vi "(RAG) Retrieve Contexts from KB.vi"(0 "Python Session Refnum in":refnum<k35>, 1 "Chroma Database Folder":path, 5 "Knowledge Base Name":string, 7 "RAG Query":string="NI 9225的最高和最低电压是多少？它的售价是多少？", 9 "K":u32=5, 11 "error in":errorcluster, 12 "Embedding Model URL":string, 13 "Embedding Model Name":string) -> (4 "Python Session Refnum out":refnum<k35>, 6 "Retrieved Contexts":string="??????∵??????? ?Ё? RoHS\n\n\n\nЁ??? National Instruments ??Ё????? ??Ё???????????? (RoHS)??? National Instruments Ё? RoHS ????????? ni.com/environment/rohs_china? (For information about China RoHS compliance, go to ni.com/ environment/rohs_china.)\n\nCalibration\n\nYou can obtain the calibration certificate and information about calibration services for the NI 9225 at ni.com/calibration.\n\nCalibration interval . 1 year\n\nWorldwide Support and Services\n??????∵??????? ?Ё? RoHS\n\n\n\nЁ??? National Instruments ??Ё????? ??Ё???????????? (RoHS)??? National Instruments Ё? RoHS ????????? ni.com/environment/rohs_china? (For information about China RoHS compliance, go to ni.com/ environment/rohs_china.)\n\nCalibration\n\nYou can obtain the calibration certificate and information about calibration services for the NI 9225 at ni.com/calibration.\n\nCalibration interval . 1 year\n\nWorldwide Support and Services\nSafety Guidelines for Hazardous Locations\n\nThe NI 9225 is suitable for use in Class I, Div 2, Gr A, B, C, D, T4 and Class I, Zn 2, Gr IIC, T4 hazardous locations, and nonhazardous locations only. Follow these guidelines if you are installing the NI 9225 in a potentially explosive environment. Not following these guidelines may result in serious injury or death.\n\nside wires or connectors d off or the area is known\nSafety Guidelines for Hazardous Locations\n\nThe NI 9225 is suitable for use in Class I, Div 2, Gr A, B, C, D, T4 and Class I, Zn 2, Gr IIC, T4 hazardous locations, and nonhazardous locations only. Follow these guidelines if you are installing the NI 9225 in a potentially explosive environment. Not following these guidelines may result in serious injury or death.\n\nside wires or connectors d off or the area is known\nchannels. NI 9225 with Conformal Coating ( ds ) 3 +/-300 V $ 3,290.00 The NI?9225 performs differential analog input. The wide measurement range is well suited for high-voltage measurement applications such as power metering, power quality monitoring, motor test, battery stack testing, and fuel cell tests. You can perform transient and harmonic analysis with high-speed simultaneous sampling. In addition, you can prevent ground loops and add safety to a system with 600?Vrms channel?to?channel", 15 "error out":errorcluster)   [LabVIEW 2023, in "LabVIEW RAG.lvlib"]
uses:
  LabVIEW RAG.lvlib
  AI RAG Globals.vi
  labview-ai-share/LabVIEW AI Base.lvlib
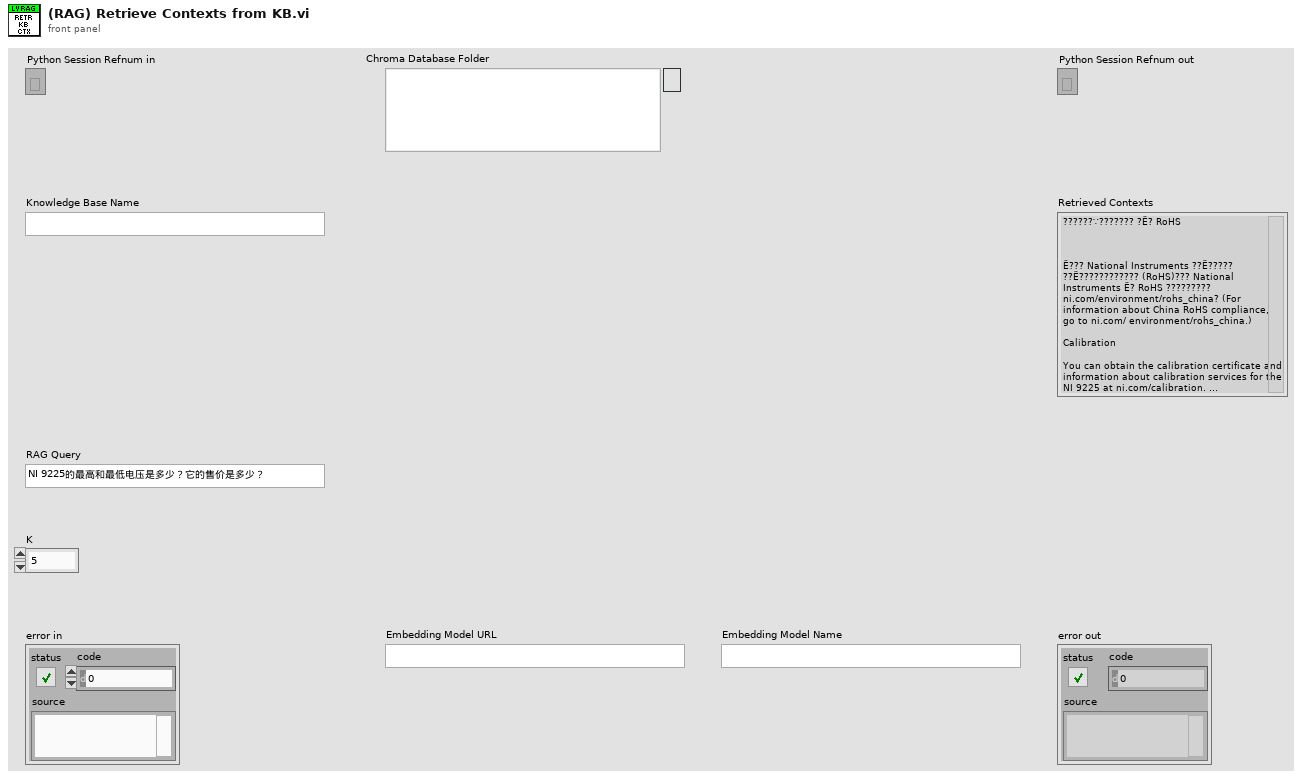
[diagram p1: front panel]
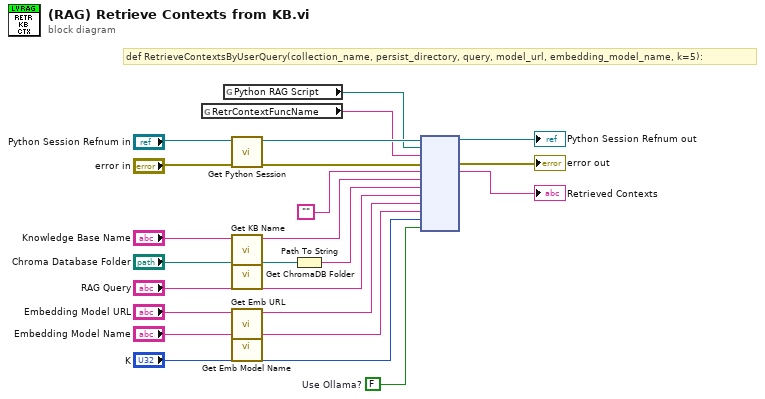
[diagram p0: block diagram]
diagram:
  w8 = FALSE  # Use Ollama?
  # "def RetrieveContextsByUserQuery(collection_name, persist_directory, query, model_url, embedding_model_name, k=5):"
  n1 = global read "AI RAG Globals.vi" "RetrContextFuncName"() -> (w5:string)
  n2 = global read "AI RAG Globals.vi" "Python RAG Script"() -> (w6:path)
  n3 = call "Get Python Session.vi"("Python Session in"="Python Session Refnum in") -> ("Python Session out"=w7:refnum<k35>)  [unwired: 10 in]
  n4 = call "Get KB Name.vi"("KB Name"="Knowledge Base Name") -> ("KB Name"=w4:string)  [unwired: 10 in]
  n5 = call "Get ChromaDB Folder.vi"("ChromaDB Folder in"="Chroma Database Folder") -> ("ChromaDB Folder out"=w3:path)  [unwired: 10 in]
  n6 = call "Get Emb URL.vi"("Embedding Model URL in"="Embedding Model URL") -> ("Embedding Model URL out"=w2:string)  [unwired: 10 in]
  n7 = call "Get Emb Model Name.vi"("Embedding Model Name in"="Embedding Model Name") -> ("Embedding Model Name out"=w1:string)  [unwired: 10 in]
  n8 = Path To String(path=w3) -> (string=w15:string)
  n9 = node(w7, w6, w5, "error in", "", w4, w15, "RAG Query", w2, w1, "K", w8) -> (→"Python Session Refnum out":refnum<k35>, →"error out":errorcluster, →"Retrieved Contexts":string)  [unwired: 7 in, 2 out]
